vi "TableScroller Original.vi"(0 "TableRef":refnum<vi>, 7 "InsertedRow":i32, 11 "#ofRows":i32) -> ()   [LabVIEW 2013]
uses:
  <vilib>/Utility/miscctls.llb/LVRowAndColumnTypeDef.ctl
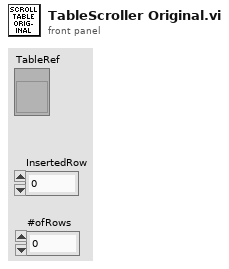
[diagram p1: front panel]
types:
  T1 = typedef "LVRowAndColumnTypeDef.ctl" = cluster{"Row":i32, "Column":i32}
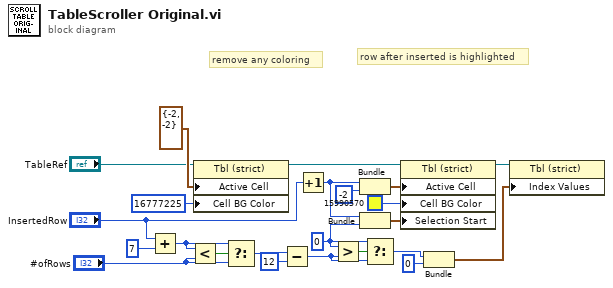
[diagram p0: block diagram]
diagram:
  w22 = 0 ("y")
  # "row after inserted is highlighted"
  # "remove any coloring"
  n1 = Add(x="InsertedRow", y=7) -> (x+y=w20:i32)
  n2 = Less?(x=w20, y="#ofRows") -> (x < y?=w4:bool)
  n3 = property on="Property Node" class="Tbl (strict)"(reference="TableRef", "Active Cell"=T1 {"Row"=-2, "Column"=-2} ("Active Cell:Active Cell"), "Cell BG Color"=u32 16777225 ("Active Cell:Cell Background Color")) -> (reference out=w14:refnum<vi>)  [unwired: 1 in, 1 out]
  n4 = Select(t=w20, s=w4, f="#ofRows") -> (s? t:f=w9:i32)
  n5 = Subtract(x=w9, y=12) -> (x-y=w7:i32)
  n6 = Increment(x="InsertedRow") -> (x+1=w21:i32)
  n7 = Greater?(x=w22, y=w7) -> (0:w6:bool)
  n8 = Bundle(w21, -2) -> (w11:cluster{i32, i32})  [unwired: 1 in]
  n9 = Bundle(w21, "y"=w22) -> (w23:cluster{i32, "y":i32})  [unwired: 1 in]
  n10 = Select(t=w22, s=w6, f=w7) -> (s? t:f=w19:i32)
  n11 = property on="Property Node" class="Tbl (strict)"(reference=w14, "Active Cell"=w11, "Cell BG Color"=u32 15990570, "Selection Start"=w23) -> (reference out=w17:refnum<vi>)  [unwired: 1 in, 1 out]
  n12 = Bundle("y"=w19, "y"=0) -> (w5:cluster{"y":i32, "y":i32})  [unwired: 1 in]
  n13 = property on="Property Node" class="Tbl (strict)"(reference=w17, "Index Values"=w5) -> ()  [unwired: 1 in, 2 out]
